vi "ReportTCPCommandTimeout.vi"(8 "error in (no error)":errorcluster, 9 "wait before close (500 ms)":u32=500, 10 "command":string, 11 "connection ID":refnum<k5>) -> (0 "error out":errorcluster, 3 "connection ID out":refnum<k5>)   [LabVIEW 2013]
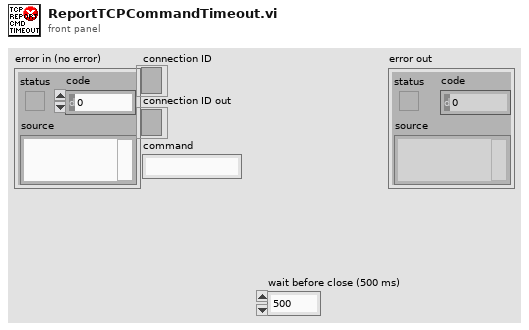
[diagram p1: front panel]
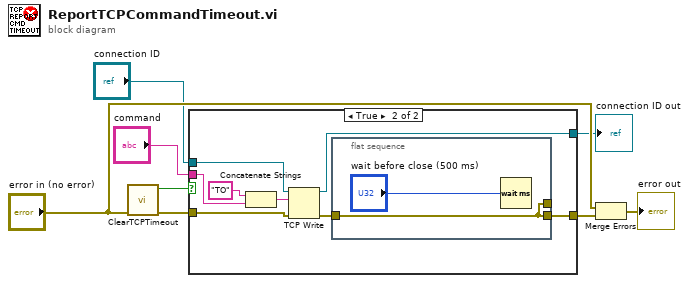
[diagram p0: block diagram]
diagram:
  n1 = call "ClearTCPTimeout.vi"("error in (no error)"="error in (no error)") -> ("error out"=w7:errorcluster, "TCP Timeout?"=w8:bool)  [unwired: 9 in]
  n2 = case shown="True" w8 {
    tunnel: w7 -> [w10 w16]
    tunnel: [w10 w12] -> w5
    tunnel: "connection ID" -> [w9 w14]
    tunnel: [w9 w15] -> w3
    tunnel: "command" -> [_ w17]
    frame False {
    }
    frame True {
      n3 = Concatenate Strings("TO" ("string"), w17) -> (w13:string)
      n4 = TCP Write(connection ID=w14, data in=w13, error in (no error)=w16) -> (connection ID out=w15:refnum<k5>, error out=w11:errorcluster)  [unwired: 1 in, 1 out]
      n5 = flat-sequence {
        tunnel: [w19] -> _
        tunnel: [w19] -> w12
        tunnel: w11 -> [w19]
        frame #0 {
          n6 = Wait (ms)(milliseconds to wait="wait before close (500 ms)") -> ()  [unwired: 1 out]
        }
      }
    }
  }
  "connection ID out" <- w3
  n7 = Merge Errors("error in (no error)", w5) -> (→"error out":errorcluster)
